vi "connect in.vi"(6 "error in (no error)":errorcluster) -> (0 "error out":errorcluster, 3 "Database Connection":T1)   [LabVIEW 2013]
doc: "Opens a connection to the database. Automatically detects if it can connect to the production database, and connects to the test database if it cannot."
uses:
  <vilib>/addons/database/Connection.llb/Conn ObjectReference.ctl
  <vilib>/addons/database/Connection.llb/DB Tools Open Connec (String).vi
  <vilib>/addons/database/NI_Database_API.lvlib
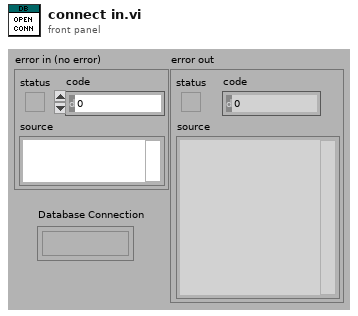
[diagram p1: front panel]
types:
  T1 = typedef "NI_Database_API.lvlib/Conn ObjectReference.ctl" = refnum<k1>
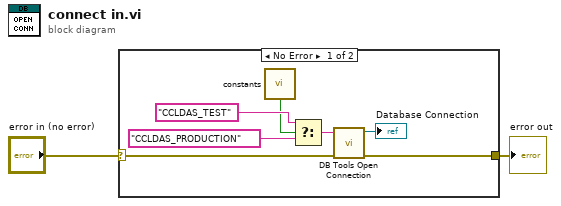
[diagram p0: block diagram]
diagram:
  n1 = case shown="No Error" "error in (no error)" {
    selector: "error in (no error)" -> [w4 w10]
    tunnel: [w8 w10] -> w1
    frame No Error {
      n2 = call "constants.vi"() -> ("Testing"=w3:bool)  [unwired: 3 in, 2 out]
      n3 = Select(t="CCLDAS_TEST", s=w3, f="CCLDAS_PRODUCTION") -> (s? t:f=w5:string)
      n4 = call-poly <vilib>:"DB Tools Open Connection.vi"("error in (no error)"=w4, "connection information"=w5) -> ("error out"=w8:errorcluster, "connection reference"=→"Database Connection":T1)  [unwired: 6 in]
    }
    frame Error {
    }
  }
  "error out" <- w1
